vi "OE2031&OE2041_Ethernet_Query Data.vi"(5 "Connection ID in":refnum<k5>, 7 "Timeout":u32=1000, 11 "Error in (no error)":errorcluster caption="error out（no error）") -> (3 "Buffer Count":u8, 4 "Connection ID out":refnum<k5>, 6 "Total Data Array":dbl[][](array[numeric]), 8 "Parameter Values":T2, 10 "Output String":string, 13 "PLL&Overload":T1, 14 "Trig In_Count":u8[](array[numeric]), 15 "Error out":errorcluster caption="error out")   [LabVIEW 2011]
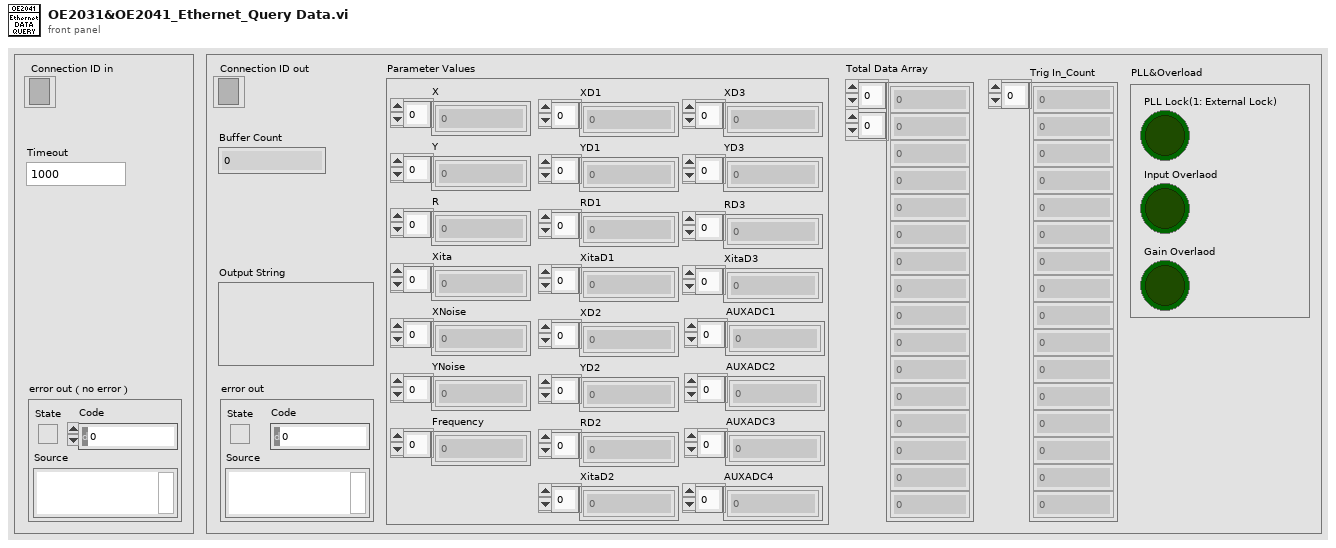
[diagram p1: front panel]
types:
  T1 = cluster{"PLL Lock(1: External Lock)":bool, "Input Overlaod":bool, "Gain Overlaod":bool}
  T2 = cluster{"X":dbl[], "Y":dbl[], "R":dbl[], "Xita":dbl[], "XNoise":dbl[], "YNoise":dbl[], "Frequency":dbl[], "XD1":dbl[], "YD1":dbl[], "RD1":dbl[], "XitaD1":dbl[], "XD2":dbl[], "YD2":dbl[], "RD2":dbl[], "XitaD2":dbl[], "XD3":dbl[], "YD3":dbl[], "RD3":dbl[], "XitaD3":dbl[], "AUXADC1":dbl[], "AUXADC2":dbl[], "AUXADC3":dbl[], "AUXADC4":dbl[]}
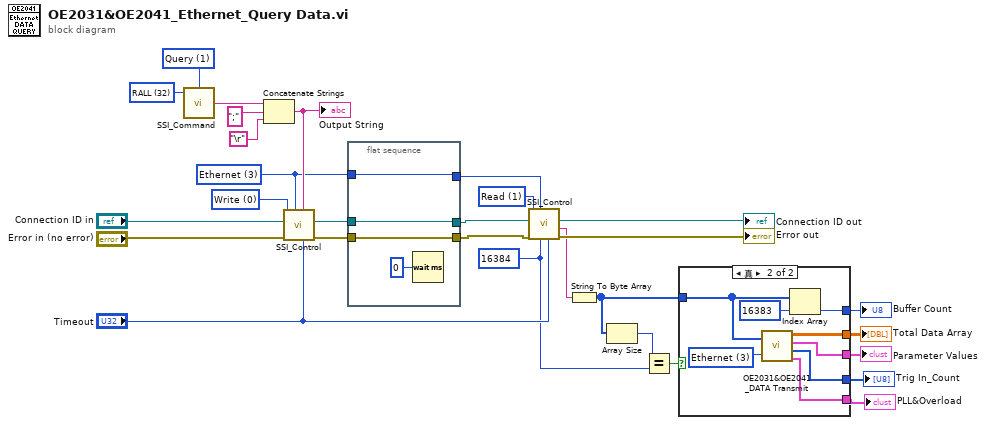
[diagram p0: block diagram]
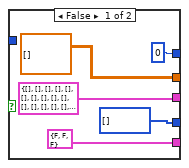
[diagram p2: hidden frame]
diagram:
  w4 = u16 3 items=["USB", "RS232", "GPIB", "Ethernet"] ("Remote Mode")
  w21 = u16 32 items=["ISRC", "IGND", "ICPL", "ILIN", "PHAS", "FMOD", "RSLP", "FREQ", "SWPT", "SLLM", "SULM", "SSLL", "SSLG", "STLM", "SWRM", "IRNG", "SENS", "RMOD", "OFLT", "OFSL", "SYNC", "DMOD", "HARM", "DARB", "SWVT", "SLVL", "SVLL", "SVUL", "SVSL", "SVSG", "SVTM", "SVRM", "RALL", "SNAP", "OUTP", "OAUX", "COUT", "CAUX", "COFP", "CEXP", "FPOP", "OEXP", "*IDN", "*RST", "OVLD", "INOV", "GNOV", "*PLL", "SSET", "RSET", "AGAN", "APHS", "ARSV", "ASCL", "EQCD", "EQCS", "SPED", "SRAT", "SLEN", "SSLE", "STRG", "SPRM", "STRD", "PAUS", "RSET", "SPTS", "TRCA", "TEMP", "RSTU", "INHZ", "DEQU", "SADD", "ARNG", "CSPE", "ISRCD", "IGNDD", "ICPLD", "ILIND", "PHASD", "FMODD", "RSLPD", "FREQD", "SWPTD", "SLLMD", "SULMD", "SSLLD", "SSLGD", "STLMD", "SWRMD", "SENSD", "RMODD", "OFLTD", "OFSLD", "SYNCD", "HARMD", "EQCDD", "EQCSD", "SNAPD", "OUTPD", "SWVTD", "SLVLD", "SVLLD", "SVULD", "SVSLD", "SVSGD", "SVTMD", "SVRMD", "SVDCD", "ARSVD", "AGAND", "APHSD", "ASCLD", "FPOPD", "CAUXD", "OEXPD", "SPEDD", "SRATD", "SLEND", "SSLED", "STRGD", "SPRMD", "STRDD", "PAUSD", "RESTD", "SPTSD", "TRCAD", "*IDND", "*RSTD", "INOVD", "GNOVD", "*PLLD", "SSETD", "RSETD", "RALLD"] ("Command Type")
  w22 = u16 1 items=["Set", "Query"] ("Opera")
  w8 = u32 16384 ("Number of bytes")
  w25 = u16 1 items=["Write", "Read"] ("Control")
  w26 = u16 0 items=["Write", "Read"] ("Control")
  n1 = call "SSI_Command.vi"("Opera"=w22, "Command Type"=w21) -> ("Output string"=w20:string)  [unwired: 2 in]
  n2 = Concatenate Strings(w20, ";" ("字符串"), "\r") -> (w23:string)
  "Output String" <- w23
  n3 = call "SSI_Control.vi"("Tineout"="Timeout", "Write Buffer"=w23, "Remote Mode"=w4, "Error in (no error)"="Error in (no error)", "Control"=w26, "Connection ID in"="Connection ID in") -> ("Error out"=w6:errorcluster, "Connection ID out"=w2:refnum<k5>)  [unwired: 2 in, 2 out]
  n4 = flat-sequence {
    tunnel: [w33] -> w5
    tunnel: w6 -> [w33]
    tunnel: [w32] -> w3
    tunnel: w4 -> [w32]
    tunnel: w2 -> [w31]
    tunnel: [w31] -> w1
    frame #0 {
      n5 = Wait (ms)(milliseconds to wait=u32 0 ("等待时间（毫秒）")) -> ()  [unwired: 1 out]
    }
  }
  n6 = call "SSI_Control.vi"("Tineout"="Timeout", "Number of bytes"=w8, "Remote Mode"=w3, "Error in (no error)"=w5, "Control"=w25, "Connection ID in"=w1) -> ("Error out"=→"Error out":errorcluster, "Read Buffer"=w17:string, "Connection ID out"=→"Connection ID out":refnum<k5>)  [unwired: 2 in, 1 out]
  n7 = String To Byte Array(string=w17) -> (unsigned byte array=w11:u8[])
  n8 = Array Size(array=w11) -> (size(s)=w10:i32)
  n9 = Equal?(x=w10, y=w8) -> (x = y?=w9:bool)
  n10 = case shown="真" w9 {
    tunnel: [u8 0 w45] -> w15
    tunnel: w11 -> [_ w44]
    tunnel: [dbl[][] [] ("Total Data Array") w42] -> w14
    tunnel: [T2 {"X"=[], "Y"=[], "R"=[], "Xita"=[], "XNoise"=[], "YNoise"=[], "Frequency"=[], "XD1"=[], "YD1"=[], "RD1"=[], "XitaD1"=[], "XD2"=[], "YD2"=[], "RD2"=[], "XitaD2"=[], "XD3"=[], "YD3"=[], "RD3"=[], "XitaD3"=[], "AUXADC1"=[], "AUXADC2"=[], "AUXADC3"=[], "AUXADC4"=[]} ("Parameter Values") w41] -> w13
    tunnel: [u8[] [] ("Trig_Count") w40] -> w12
    tunnel: [T1 {"PLL Lock(1: External Lock)"=FALSE, "Input Overlaod"=FALSE, "Gain Overlaod"=FALSE} ("PLL&Overload") w39] -> w7
    frame False {
    }
    frame True {
      w43 = u16 3 items=["USB"=0, "Ethernet"=3] ("Remote Mode")
      n11 = call "OE2031&OE2041_DATA Transmit.vi"("Input Data"=w44, "Remote Mode"=w43) -> ("Total Data Array"=w42:dbl[][], "Parameter Values"=w41:T2, "Trig_Count"=w40:u8[], "PLL&Overload"=w39:T1)
      n12 = Index Array(array=w44, index=16383 ("索引")) -> (element=w45:u8)
    }
  }
  "Parameter Values" <- w13
  "Total Data Array" <- w14
  "Buffer Count" <- w15
  "Trig In_Count" <- w12
  "PLL&Overload" <- w7
